vi "LCP Configure Conti Flow Valve.vi"(6 "ValveIndex":u32, 7 "PumpChannelIndex":u32, 8 "error in (no error)":errorcluster caption="Fehler (Eingang, kein Fehler)", 10 "ValveConfig":T1, 11 "ContiFlowPumpHandle":i64) -> (0 "error out":errorcluster caption="Fehler (Ausgang)", 3 "ContiFlowPumpHandle Out":i64)   [LabVIEW 2021, in "labbCAN_Pump_API.lvlib"]
uses:
  labbCAN_Pump_API.lvlib
  labbCAN_Pump_API.dll
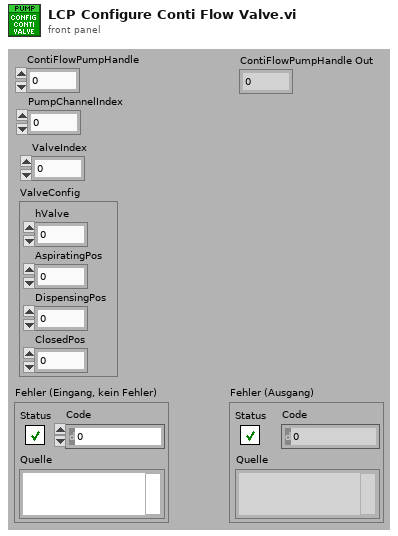
[diagram p1: front panel]
types:
  T1 = cluster{"hValve":i64, "AspiratingPos":i32, "DispensingPos":i32, "ClosedPos":i32}
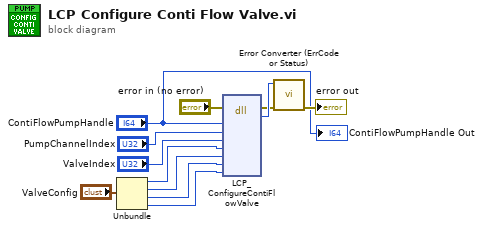
[diagram p0: block diagram]
diagram:
  n1 = Unbundle("ValveConfig") -> ("hValve"=w5:i64, "AspiratingPos"=w4:i32, "DispensingPos"=w3:i32, "ClosedPos"=w2:i32)
  n2 = dll-call lib="C:/Users/olaja/AppData/Local/CETONI_SDK/labbCAN_Pump_API.*" fn="LCP_ConfigureContiFlowValve"(error in="error in (no error)", "hContiFlowPump"="ContiFlowPumpHandle", "PumpChannelIndex"="PumpChannelIndex", "ValveIndex"="ValveIndex", "hValve"=w5, "AspiratingPos"=w4, "DispensingPos"=w3, "ClosedPos"=w2) -> (error out=w10:errorcluster, "Rückgabetyp"=w12:i32)  [unwired: 9 in, 1 out]
  n3 = call "Error Converter (ErrCode or Status).vi"("error in (no error)"=w10, "error code"=w12) -> ("error out"=→"error out":errorcluster)  [unwired: 9 in]
  "ContiFlowPumpHandle Out" <- "ContiFlowPumpHandle"
